vi "OPC UA Server.vi"() -> (0 "error out":errorcluster)   [LabVIEW 2021, in "OPC UA Server.lvlib"]
doc: "Use this template to build a simple state machine design pattern. Each state executes code and determines which state to transition to."
uses:
  OPC UA Server.lvlib
  Rx from PLC.ctl
  Tx to PLC.ctl
  State.ctl
  Local Dataset.ctl
  <vilib>/OPCUA/controls/OPC UA Server Refnum.ctl
  <vilib>/OPCUA/controls/Supported Security Policies.ctl
  <vilib>/OPCUA/controls/Data Type.ctl
  <vilib>/OPCUA/server/Read Variant.vi
  <vilib>/OPCUA/server/Write Variant.vi
  <vilib>/OPCUA/NI OPC UA Server.lvlib
panel:
  in  "Initialization":bool
  out "StationB Tester Tx":T1
  in  "StationB Tester Rx":T2={"Start"=TRUE, "NestStatus"=TRUE, "PalletID"=1, "BarcodeData"="P:S", "StepEcho"=4, "Cylinder_1"=TRUE, "Cylinder_2"=FALSE, "Cylinder_3"=FALSE, "Cylinder_4"=TRUE, "Cylinder_5"=TRUE, "ResultsAck"=TRUE, "Reset"=FALSE, "Stop"=FALSE, "FaultCode"=0}
  in  "Folder names":string[](array[string])=["StaARx#[PLC]StaATesterRxSignals", "StaATx#[PLC]StaATesterTxSignals", "StaBRx#[PLC]StaBTesterRxSignals", "StaBTx#[PLC]StaBTesterTxSignals"]
  out "StationA Tester Tx":T1
  in  "StationA Tester Rx":T2={"Start"=TRUE, "NestStatus"=TRUE, "PalletID"=1, "BarcodeData"="P:S", "StepEcho"=4, "Cylinder_1"=TRUE, "Cylinder_2"=FALSE, "Cylinder_3"=FALSE, "Cylinder_4"=TRUE, "Cylinder_5"=TRUE, "ResultsAck"=TRUE, "Reset"=FALSE, "Stop"=FALSE, "FaultCode"=0}
  out "Network":bool
  out "server endpoint URL":string="opc.tcp://JLee-Laptop:49580"
  # "MM, DD, YY. hh, mm, ss, ms"
  # "MM, DD, YY. hh, mm, ss, ms"
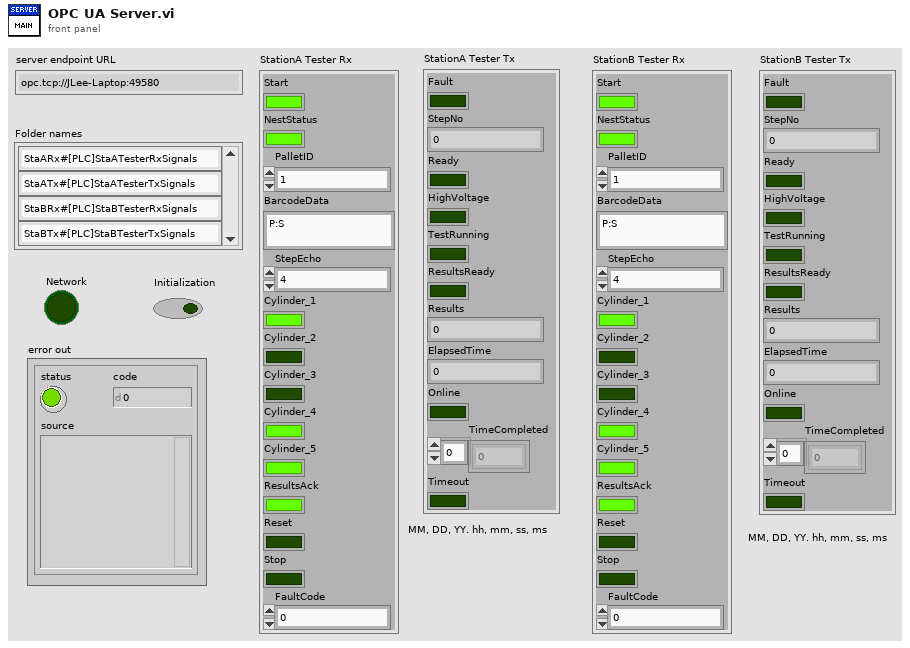
[diagram p1: front panel]
types:
  T1 = typedef "OPC UA Server.lvlib/Tx to PLC.ctl" = cluster{"Fault":bool, "StepNo":i32, "Ready":bool, "HighVoltage":bool, "TestRunning":bool, "ResultsReady":bool, "Results":i32, "ElapsedTime":i32, "Online":bool, "TimeCompleted":i32[], "Timeout":bool}
  T2 = typedef "OPC UA Server.lvlib/Rx from PLC.ctl" = cluster{"Start":bool, "NestStatus":bool, "PalletID":i32, "BarcodeData":string, "StepEcho":u32, "Cylinder_1":bool, "Cylinder_2":bool, "Cylinder_3":bool, "Cylinder_4":bool, "Cylinder_5":bool, "ResultsAck":bool, "Reset":bool, "Stop":bool, "FaultCode":i32}
  T3 = typedef "Supported Security Policies.ctl" = cluster{"None":bool, "Sign with Basic128Rsa15":bool, "Sign and Encrypt with Basic128Rsa15":bool, "Sign with Basic256":bool, "Sign and Encrypt with Basic256":bool}
  T4 = typedef "OPC UA Server.lvlib/Local Dataset.ctl" = cluster{"OPC server":T5, "Tag ItemIDs":string[][], "StationA Tester Rx":refnum<vi>, "StationA Tester Tx":refnum<vi>, "StationB Tester Rx":refnum<vi>, "StationB Tester Tx":refnum<vi>, "Folder NodeIDs":string[]}
  T5 = typedef "OPC UA Server Refnum.ctl" = refnum<k21>
  T6 = typedef "OPC UA Server.lvlib/State.ctl" = enum16{"Initialize", "Config", "Wait for Event", "Exit"}
  T7 = typedef "Data Type.ctl" = u16
  T8 = cluster{"name":string, "data type":T7, "access level":u16, "description":string}
  T9 = typedef "NodeId.ctl" = string
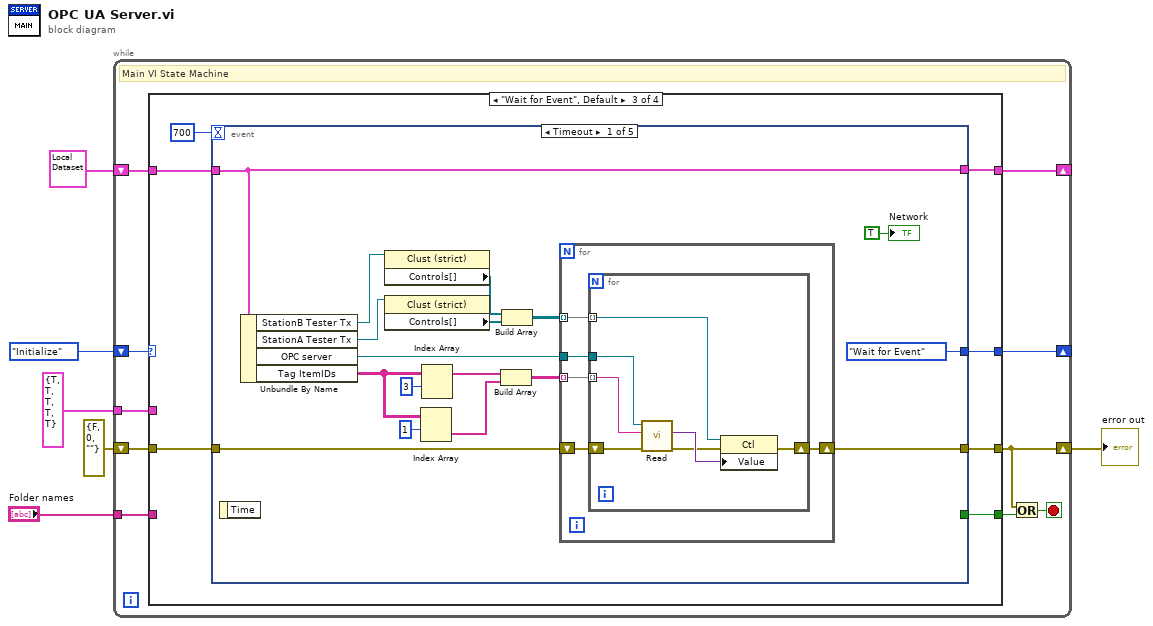
[diagram p0: block diagram]
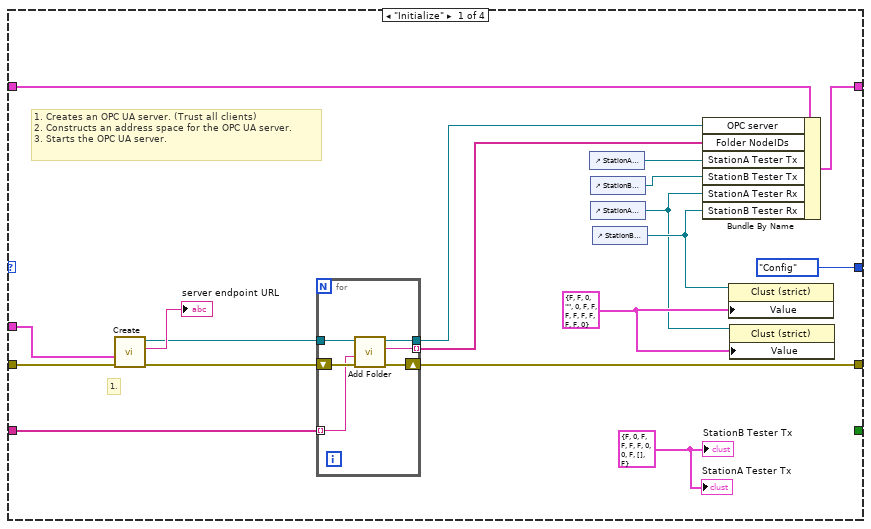
[diagram p2: hidden frame]
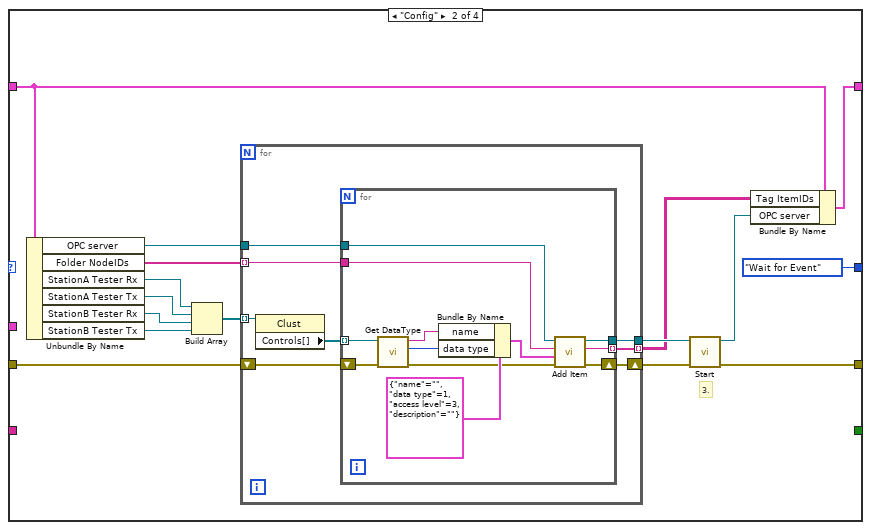
[diagram p3: hidden frame]
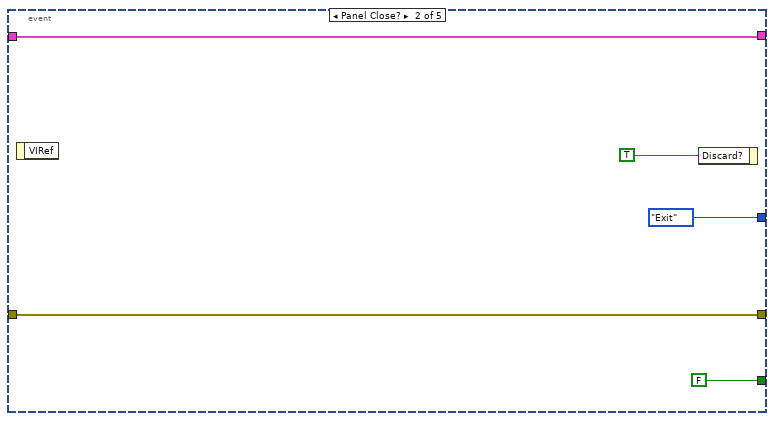
[diagram p4: hidden frame]
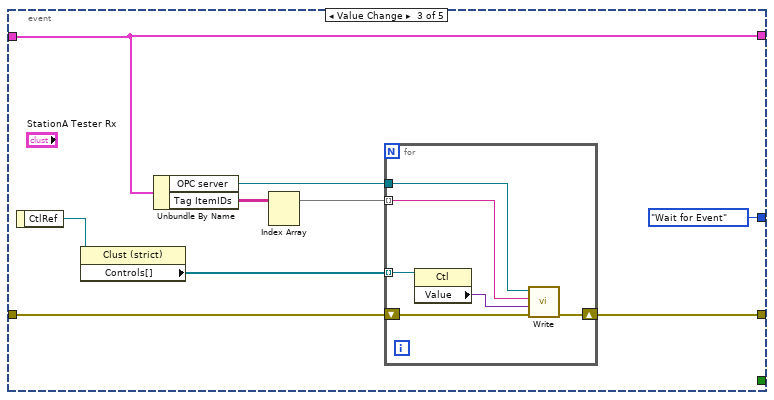
[diagram p5: hidden frame]
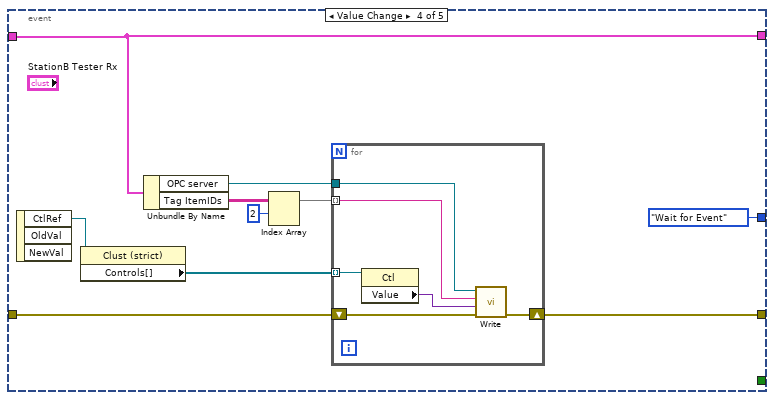
[diagram p6: hidden frame]
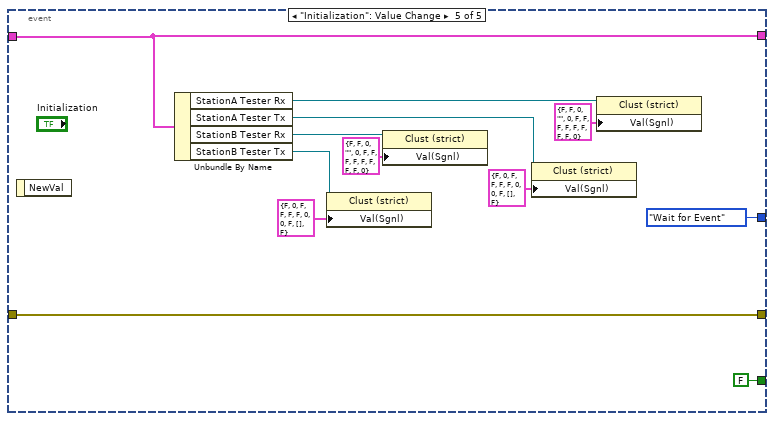
[diagram p7: hidden frame]
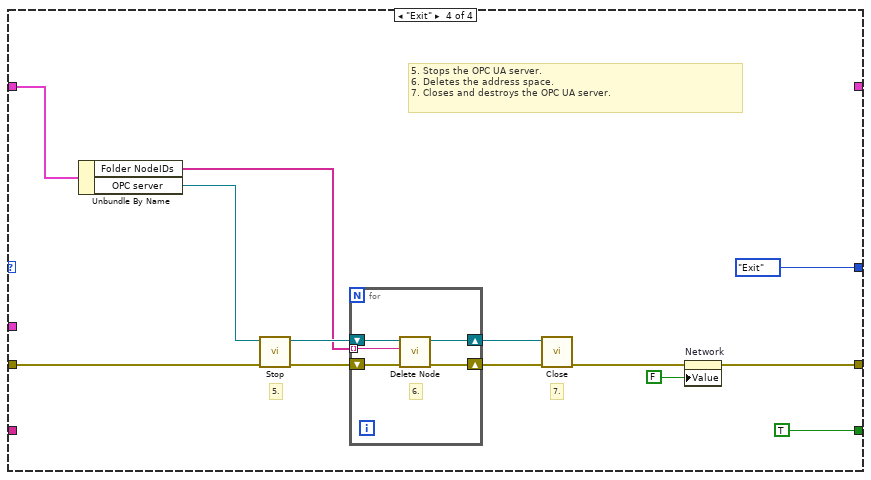
[diagram p8: hidden frame]
diagram:
  n1 = while {
    shift-right: [w15] -> _
    shift-left: State."Initialize" ("Initial State") -> [w16]
    shift-right: [w13] -> _
    shift-left: T4 {"OPC server"="", "Tag ItemIDs"=[], "StationA Tester Rx"=refnum, "StationA Tester Tx"=refnum, "StationB Tester Rx"=refnum, "StationB Tester Tx"=refnum, "Folder NodeIDs"=[]} ("Data") -> [w14]
    shift-right: [w9] -> w1
    shift-left: errorcluster {"status"=FALSE, "code"=0, "source"=""} ("error out") -> [w12]
    tunnel: T3 {"None"=TRUE, "Sign with Basic128Rsa15"=TRUE, "Sign and Encrypt with Basic128Rsa15"=TRUE, "Sign with Basic256"=TRUE, "Sign and Encrypt with Basic256"=TRUE} ("supported security policies (None)") -> [w8]
    tunnel: "Folder names" -> [w7]
    stop <- w10 stop-if-true
    # "Main VI State Machine"
    n2 = case shown="\"Wait for Event\", Default" w16 {
      tunnel: [State."Config" ("Next State") State."Wait for Event" ("(Value Not Used)") w82 State."Exit" ("(Value Not Used)")] -> w15
      tunnel: [_ _ w83 TRUE ("Stop Loop?")] -> w11
      tunnel: w14 -> [w29 w55 w78 w166]
      tunnel: [w33 w56 w81 _] -> w13
      tunnel: w12 -> [w32 w43 w77 w167]
      tunnel: [w24 w45 w80 w161] -> w9
      tunnel: w8 -> [w23 _ _ _]
      tunnel: w7 -> [w25 _ _ _]
      frame "Initialize" {
        w21 = T2 {"Start"=FALSE, "NestStatus"=FALSE, "PalletID"=0, "BarcodeData"="", "StepEcho"=0, "Cylinder_1"=FALSE, "Cylinder_2"=FALSE, "Cylinder_3"=FALSE, "Cylinder_4"=FALSE, "Cylinder_5"=FALSE, "ResultsAck"=FALSE, "Reset"=FALSE, "Stop"=FALSE, "FaultCode"=0} ("Rx from PLC")
        w22 = T1 {"Fault"=FALSE, "StepNo"=0, "Ready"=FALSE, "HighVoltage"=FALSE, "TestRunning"=FALSE, "ResultsReady"=FALSE, "Results"=0, "ElapsedTime"=0, "Online"=FALSE, "TimeCompleted"=[], "Timeout"=FALSE} ("Rx from Tester")
        # "1. Creates an OPC UA server. (Trust all clients)\n2. Constructs an address space for the OPC UA server.\n3. Starts the OPC UA server."
        # "1."
        # "Initialize - Initialize the application."
        n3 = call <vilib>:"Create.vi"("error in (no error)"=w32, "supported security policies (None)"=w23) -> ("error out"=w31:errorcluster, "server endpoint URL"=→"server endpoint URL":string, "OPC UA server refnum out"=w28:T5)  [unwired: 7 in]
        n4 = for {
          tunnel: [w37] -> w26 mode=indexing
          tunnel: w25 -> [w36] mode=indexing
          shift-right: [w35] -> w24
          shift-left: w31 -> [w40]
          tunnel: w28 -> [w39]
          tunnel: [w38] -> w27
          n5 = call <vilib>:"Add Folder.vi"("error in (no error)"=w40, "folder name"=w36, "OPC UA server refnum in"=w39) -> ("error out"=w35:errorcluster, "folder node ID"=w37:T9, "OPC UA server refnum out"=w38:T5)  [unwired: 5 in]
        }
        n6 = control-ref of="StationA Tester Tx"() -> (w17:refnum<vi>)
        n7 = control-ref of="StationB Tester Tx"() -> (w18:refnum<vi>)
        n8 = control-ref of="StationA Tester Rx"() -> (w19:refnum<vi>)
        n9 = control-ref of="StationB Tester Rx"() -> (w20:refnum<vi>)
        n10 = Bundle By Name(cluster=w29, "OPC server"=w27, "Folder NodeIDs"=w26, "StationA Tester Tx"=w17, "StationB Tester Tx"=w18, "StationA Tester Rx"=w19, "StationB Tester Rx"=w20) -> (w33:T4)
        n11 = property class="Clust (strict)"(reference=w20, "Value"=w21) -> ()  [unwired: 1 in, 2 out]
        n12 = property class="Clust (strict)"(reference=w19, "Value"=w21) -> ()  [unwired: 1 in, 2 out]
        "StationA Tester Tx" <- w22
        "StationB Tester Tx" <- w22
      }
      frame "Config" {
        # "3."
        n13 = Unbundle By Name(w55) -> ("OPC server"=w50:T5, "Folder NodeIDs"=w53:string[], "StationA Tester Rx"=w48:refnum<vi>, "StationA Tester Tx"=w47:refnum<vi>, "StationB Tester Rx"=w42:refnum<vi>, "StationB Tester Tx"=w41:refnum<vi>)
        n14 = Build Array(w48, w47, w42, w41) -> (w46:refnum<vi>[])
        n15 = for {
          tunnel: w53 -> [w63] mode=indexing
          tunnel: [w59] -> w49 mode=indexing
          tunnel: w46 -> [w58] mode=indexing
          shift-right: [w62] -> w44
          shift-left: w43 -> [w64]
          tunnel: w50 -> [w60]
          tunnel: [w61] -> w51
          n16 = property class="Clust"(reference=w58) -> ("Controls[]"=w57:refnum<vi>[])  [unwired: 1 in, 2 out]
          n17 = for {
            tunnel: w60 -> [w76]
            tunnel: w63 -> [w75]
            tunnel: [w73] -> w61
            shift-right: [w74] -> w62
            shift-left: w64 -> [w68]
            tunnel: [w72] -> w59 mode=indexing
            tunnel: w57 -> [w69] mode=indexing
            n18 = call "Get DataType.vi"("error in (no error)"=w68, "reference"=w69) -> ("error out"=w66:errorcluster, "data type"=w65:T7, "Name"=w67:string)  [unwired: 7 in]
            n19 = Bundle By Name(cluster=T8 {"name"="", "data type"=1, "access level"=3, "description"=""} ("item"), "name"=w67, "data type"=w65) -> (w70:T8)
            n20 = call <vilib>:"Add Item.vi"("error in (no error)"=w66, "item"=w70, "parent folder node ID"=w75, "OPC UA server refnum in"=w76) -> ("error out"=w74:errorcluster, "item node ID"=w72:T9, "OPC UA server refnum out"=w73:T5)  [unwired: 3 in, 1 out]
          }
        }
        n21 = call <vilib>:"Start.vi"("error in (no error)"=w44, "OPC UA server refnum in"=w51) -> ("error out"=w45:errorcluster, "OPC UA server refnum out"=w54:T5)  [unwired: 7 in, 1 out]
        n22 = Bundle By Name(cluster=w55, "Tag ItemIDs"=w49, "OPC server"=w54) -> (w56:T4)
      }
      frame "Wait for Event", Default {
        # "Wait for Event - Use an Event Structure to monitor the user interface for events that run different states of the state machine."
        n23 = event shown="[0] Timeout" {
          selector: _ -> [_ _ _ _ _]
          dyn-events: _ -> [_ _ _ _ _]
          timeout: 700 -> [_ _ _ _ _]
          tunnel: [_ FALSE ("NewVal") _ _ FALSE ("NewVal")] -> w83
          tunnel: [State."Wait for Event" ("(Value Not Used)") State."Exit" ("(Value Not Used)") State."Wait for Event" ("(Value Not Used)") State."Wait for Event" ("(Value Not Used)") State."Wait for Event" ("(Value Not Used)")] -> w82
          tunnel: w78 -> [w100 w116 w125 w141 w160]
          tunnel: [w100 w116 w125 w141 w160] -> w81
          tunnel: w77 -> [w96 w114 w122 w138 w151]
          tunnel: [w95 w114 w124 w140 w151] -> w80
          event Timeout {
            n24 = event-data() -> ()  [unwired: 1 in, 1 out]
            n25 = Unbundle By Name(w100) -> ("StationB Tester Tx"=w92:refnum<vi>, "StationA Tester Tx"=w94:refnum<vi>, "OPC server"=w97:T5, "Tag ItemIDs"=w90:string[][])
            n26 = property class="Clust (strict)"(reference=w92) -> ("Controls[]"=w89:refnum<vi>[])  [unwired: 1 in, 2 out]
            n27 = property class="Clust (strict)"(reference=w94) -> ("Controls[]"=w88:refnum<vi>[])  [unwired: 1 in, 2 out]
            n28 = Index Array(array=w90, index (row)=1) -> (element=w86:string[])  [unwired: 1 in]
            n29 = Index Array(array=w90, index (row)=3) -> (element=w87:string[])  [unwired: 1 in]
            n30 = Build Array(w87, w86) -> (w85:string[][])
            n31 = Build Array(w89, w88) -> (w84:refnum<vi>[][])
            n32 = for {
              tunnel: w97 -> [w105]
              tunnel: w85 -> [w102] mode=indexing
              shift-right: [w103] -> w95
              shift-left: w96 -> [w104]
              tunnel: w84 -> [w101] mode=indexing
              n33 = for {
                tunnel: w105 -> [w110]
                tunnel: w101 -> [w112] mode=indexing
                shift-right: [w106] -> w103
                shift-left: w104 -> [w111]
                tunnel: w102 -> [w109] mode=indexing
                n34 = call-poly <vilib>:"Read.vi"("error in (no error)"=w111, "node ID"=w109, "OPC UA server refnum in"=w110) -> ("error out"=w107:errorcluster, "value"=w108:variant)  [unwired: 4 in, 3 out]
                n35 = property class="Ctl"(reference=w112, error in=w107, "Value"=w108) -> (error out=w106:errorcluster)  [unwired: 1 out]
              }
            }
            "Network" <- TRUE ("Network")
          }
          event Panel Close? {
            n36 = event-data() -> ()  [unwired: 1 in, 1 out]
            n37 = event-data("Discard?"=TRUE) -> ()  [unwired: 1 in, 1 out]
          }
          event Value Change {
            n38 = event-data() -> ("CtlRef"=w120:refnum<vi>)  [unwired: 1 in]
            n39 = property class="Clust (strict)"(reference=w120) -> ("Controls[]"=w119:refnum<vi>[])  [unwired: 1 in, 2 out]
            n40 = Unbundle By Name(w125) -> ("OPC server"=w126:T5, "Tag ItemIDs"=w121:string[][])
            n41 = Index Array(array=w121) -> (element=w118:string[])  [unwired: 2 in]
            n42 = for {
              tunnel: w126 -> [w132]
              tunnel: w119 -> [w128] mode=indexing
              shift-right: [w131] -> w124
              shift-left: w122 -> [w130]
              tunnel: w118 -> [w129] mode=indexing
              n43 = property class="Ctl"(reference=w128) -> ("Value"=w127:variant)  [unwired: 1 in, 2 out]
              n44 = call-poly <vilib>:"Write.vi"("error in (no error)"=w130, "value"=w127, "node ID"=w129, "OPC UA server refnum in"=w132) -> ("error out"=w131:errorcluster)  [unwired: 5 in, 2 out]
            }
          }
          event Value Change {
            n45 = event-data() -> ("CtlRef"=w136:refnum<vi>)  [unwired: 1 in, 2 out]
            n46 = property class="Clust (strict)"(reference=w136) -> ("Controls[]"=w135:refnum<vi>[])  [unwired: 1 in, 2 out]
            n47 = Unbundle By Name(w141) -> ("OPC server"=w142:T5, "Tag ItemIDs"=w137:string[][])
            n48 = Index Array(array=w137, index (row)=2) -> (element=w134:string[])  [unwired: 1 in]
            n49 = for {
              tunnel: w142 -> [w148]
              tunnel: w135 -> [w144] mode=indexing
              shift-right: [w147] -> w140
              shift-left: w138 -> [w146]
              tunnel: w134 -> [w145] mode=indexing
              n50 = property class="Ctl"(reference=w144) -> ("Value"=w143:variant)  [unwired: 1 in, 2 out]
              n51 = call-poly <vilib>:"Write.vi"("error in (no error)"=w146, "value"=w143, "node ID"=w145, "OPC UA server refnum in"=w148) -> ("error out"=w147:errorcluster)  [unwired: 5 in, 2 out]
            }
          }
          event "Initialization": Value Change {
            n52 = event-data() -> ()  [unwired: 1 in, 1 out]
            n53 = Unbundle By Name(w160) -> ("StationA Tester Rx"=w159:refnum<vi>, "StationA Tester Tx"=w157:refnum<vi>, "StationB Tester Rx"=w153:refnum<vi>, "StationB Tester Tx"=w152:refnum<vi>)
            n54 = property class="Clust (strict)"(reference=w152, "Val(Sgnl)"=T1 {"Fault"=FALSE, "StepNo"=0, "Ready"=FALSE, "HighVoltage"=FALSE, "TestRunning"=FALSE, "ResultsReady"=FALSE, "Results"=0, "ElapsedTime"=0, "Online"=FALSE, "TimeCompleted"=[], "Timeout"=FALSE} ("Tx to PLC")) -> ()  [unwired: 1 in, 2 out]
            n55 = property class="Clust (strict)"(reference=w153, "Val(Sgnl)"=T2 {"Start"=FALSE, "NestStatus"=FALSE, "PalletID"=0, "BarcodeData"="", "StepEcho"=0, "Cylinder_1"=FALSE, "Cylinder_2"=FALSE, "Cylinder_3"=FALSE, "Cylinder_4"=FALSE, "Cylinder_5"=FALSE, "ResultsAck"=FALSE, "Reset"=FALSE, "Stop"=FALSE, "FaultCode"=0} ("Rx from PLC")) -> ()  [unwired: 1 in, 2 out]
            n56 = property class="Clust (strict)"(reference=w157, "Val(Sgnl)"=T1 {"Fault"=FALSE, "StepNo"=0, "Ready"=FALSE, "HighVoltage"=FALSE, "TestRunning"=FALSE, "ResultsReady"=FALSE, "Results"=0, "ElapsedTime"=0, "Online"=FALSE, "TimeCompleted"=[], "Timeout"=FALSE} ("Tx to PLC")) -> ()  [unwired: 1 in, 2 out]
            n57 = property class="Clust (strict)"(reference=w159, "Val(Sgnl)"=T2 {"Start"=FALSE, "NestStatus"=FALSE, "PalletID"=0, "BarcodeData"="", "StepEcho"=0, "Cylinder_1"=FALSE, "Cylinder_2"=FALSE, "Cylinder_3"=FALSE, "Cylinder_4"=FALSE, "Cylinder_5"=FALSE, "ResultsAck"=FALSE, "Reset"=FALSE, "Stop"=FALSE, "FaultCode"=0} ("Rx from PLC")) -> ()  [unwired: 1 in, 2 out]
          }
        }
      }
      frame "Exit" {
        # "5."
        # "5. Stops the OPC UA server.\n6. Deletes the address space.\n7. Closes and destroys the OPC UA server."
        # "7."
        # "Exit - Exit the application."
        n58 = Unbundle By Name(w166) -> ("Folder NodeIDs"=w164:string[], "OPC server"=w165:T5)
        n59 = call <vilib>:"Stop.vi"("error in (no error)"=w167, "OPC UA server refnum in"=w165) -> ("error out"=w171:errorcluster, "OPC UA server refnum out"=w170:T5)  [unwired: 8 in]
        n60 = for {
          tunnel: w164 -> [w174] mode=indexing
          shift-right: [w176] -> w169
          shift-left: w171 -> [w178]
          shift-right: [w175] -> w168
          shift-left: w170 -> [w177]
          # "6."
          n61 = call <vilib>:"Delete Node.vi"("error in (no error)"=w178, "node ID"=w174, "OPC UA server refnum in"=w177) -> ("error out"=w176:errorcluster, "OPC UA server refnum out"=w175:T5)  [unwired: 7 in]
        }
        n62 = call <vilib>:"Close.vi"("error in (no error)"=w169, "OPC UA server refnum in"=w168) -> ("error out"=w162:errorcluster)  [unwired: 9 in]
        n63 = property on="Network" class="Bool (strict)"(error in=w162, "Value"=FALSE ("Network")) -> (error out=w161:errorcluster)  [unwired: 1 in, 1 out]
      }
    }
    n64 = Or(x=w9, y=w11) -> (x .or. y?=w10:bool)
  }
  "error out" <- w1
